vi "Get DDG Pulse.vi"(7 "Width":dbl, 9 "Delay":dbl, 10 "resolution":dbl, 11 "wid":dbl) -> (1 "Delay out":dbl, 3 "function return":u32, 5 "Width out":dbl)   [LabVIEW 2018, in "AndorSDK.lvlib"]
doc: "EXPNETTYPE unsigned int WINAPI GetDDGPulse(double wid, double resolution, double * Delay, double * Width);"
uses:
  AndorSDK.lvlib
  ATMCD32D.dll
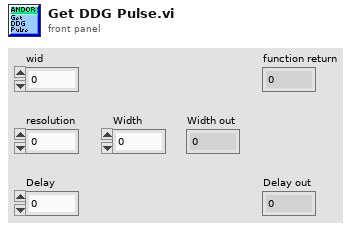
[diagram p1: front panel]
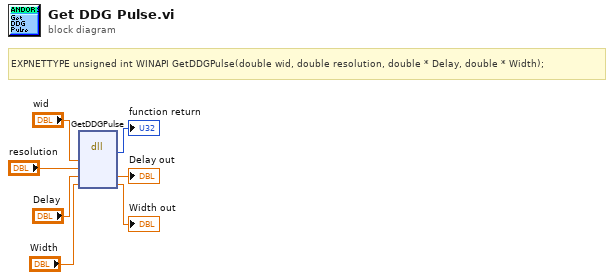
[diagram p0: block diagram]
diagram:
  # "EXPNETTYPE unsigned int WINAPI GetDDGPulse(double wid, double resolution, double * Delay, double * Width);"
  n1 = dll-call lib="PTH2babs E\nPersönliches02 - Arbeit03-HiwijobsLabviewCodelibANDOR\tAndor SDK\nATMCD32D.*" fn="GetDDGPulse"("wid"="wid", "resolution"="resolution", "Delay"="Delay", "Width"="Width") -> (→"function return":u32, "Delay"=→"Delay out":dbl, "Width"=→"Width out":dbl)  [unwired: 5 in, 2 out]
